vi "Signal Manipulations.vi"(4 "INPUT1 Differential Mode":bool, 5 "VDC INPUT2":dbl, 6 "INPUT2 Differential Mode":bool, 7 "VDC INPUT1":dbl, 8 "INPUT 2R Loc":dbl min=-450.0 max=450.0 step=0.001, 9 "INPUT 2R Line In":dbl[](graph), 10 "INPUT 1L Loc":dbl min=-450.0 max=450.0 step=0.001, 11 "INPUT 1L Line In":dbl[](graph)) -> (0 "VDC INPUT2":dbl, 1 "VDC INPUT1":dbl, 2 "INPUT1L Line Out":dbl[](graph), 3 "INPUT2R Line Out":dbl[](graph))   [LabVIEW 2012]
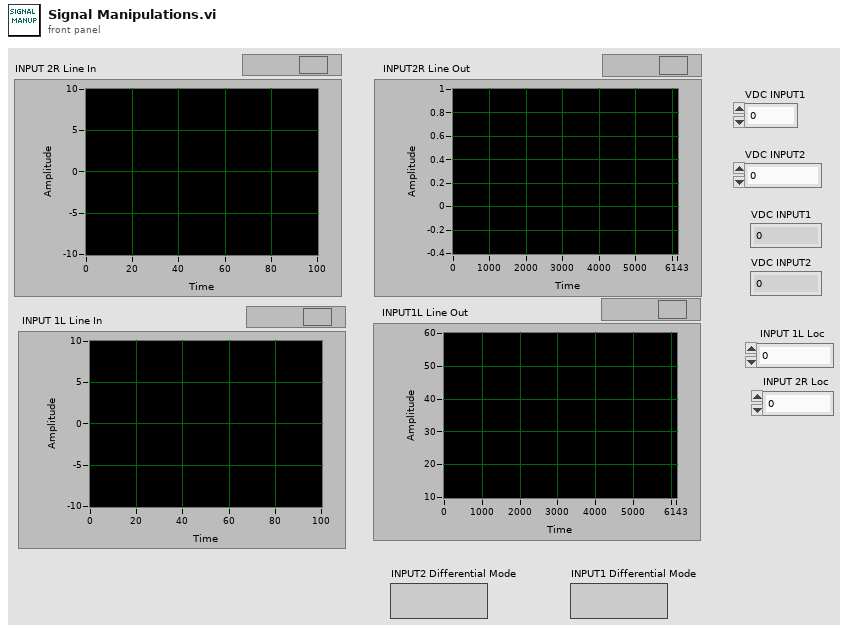
[diagram p1: front panel]
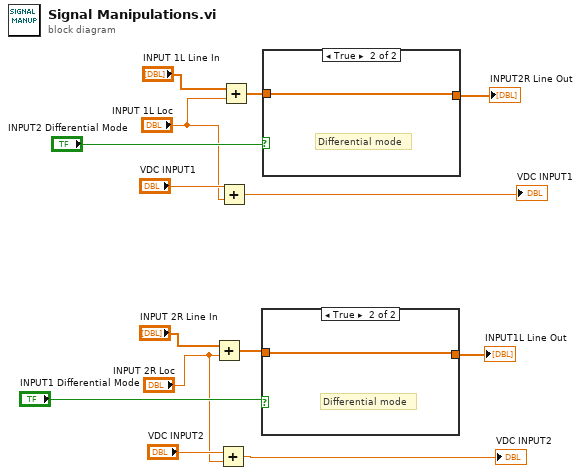
[diagram p0: block diagram]
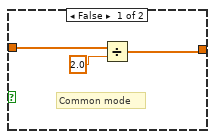
[diagram p2: hidden frame]
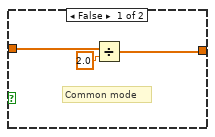
[diagram p3: hidden frame]
diagram:
  n1 = Add(x="INPUT 2R Line In", y="INPUT 2R Loc") -> (x+y=w9:dbl[])
  n2 = Add(x="VDC INPUT2", y="INPUT 2R Loc") -> (x+y=→"VDC INPUT2":dbl)
  n3 = Add(x="VDC INPUT1", y="INPUT 1L Loc") -> (x+y=→"VDC INPUT1":dbl)
  n4 = Add(x="INPUT 1L Line In", y="INPUT 1L Loc") -> (x+y=w12:dbl[])
  n5 = case shown="True" "INPUT1 Differential Mode" {
    tunnel: [w17 w18] -> w8
    tunnel: w9 -> [w16 w18]
    frame False {
      # "Common mode"
      n6 = Divide(x=w16, y=2.0) -> (x/y=w17:dbl[])
    }
    frame True {
      # "Differential mode"
    }
  }
  "INPUT1L Line Out" <- w8
  n7 = case shown="True" "INPUT2 Differential Mode" {
    tunnel: [w21 w22] -> w11
    tunnel: w12 -> [w20 w22]
    frame False {
      # "Common mode"
      n8 = Divide(x=w20, y=2.0) -> (x/y=w21:dbl[])
    }
    frame True {
      # "Differential mode"
    }
  }
  "INPUT2R Line Out" <- w11
